vi "Evaluate Observables.vi"(8 "error in (no error)":errorcluster, 9 "Observables with values":T3[](array[typedef]), 10 "Obsv to check":T2(array[cluster]), 11 "Analysis Framework in":refnum<class "Analysis Framework.lvclass">) -> (0 "error out":errorcluster, 2 "Evaluation":T1, 3 "Analysis Framework out":refnum<class "Analysis Framework.lvclass">)   [LabVIEW 2020, in "Analysis Framework.lvclass"]
uses:
  Analysis Framework.lvclass
  Run Utilities/Optimiser Cell/Name with value pair.ctl
  Run Utilities/TypeDefs/Return Code.ctl
  Run Utilities/Run Utilities.lvlib
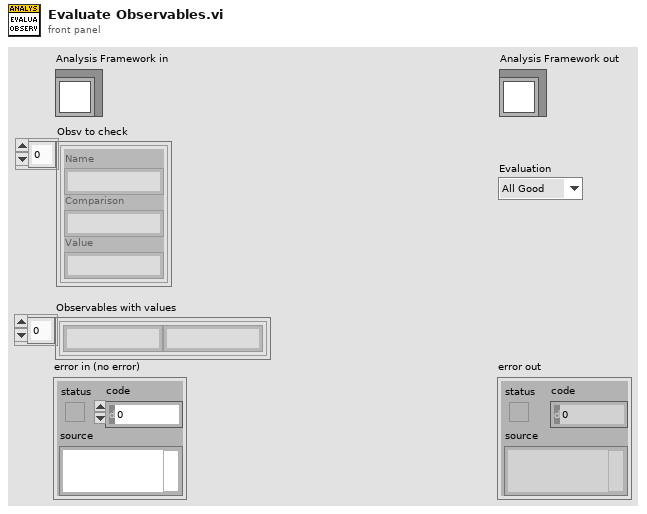
[diagram p1: front panel]
types:
  T1 = typedef "Run Utilities.lvlib/Return Code.ctl" = enum16{"All Good", "Retry", "Skip", "Skip All", "ABORT"}
  T2 = cluster{"Name":string, "Comparison":string, "Value":string}[]
  T3 = typedef "Analysis Framework.lvclass/Name with value pair.ctl" = cluster{"Name":string, "Value":string}
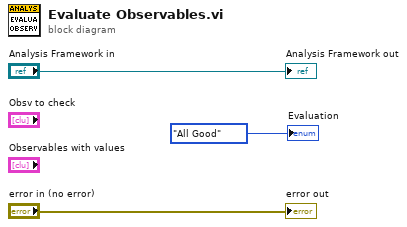
[diagram p0: block diagram]
diagram:
  "error out" <- "error in (no error)"
  "Analysis Framework out" <- "Analysis Framework in"
  "Evaluation" <- Return_Code."All Good" ("Evaluation")
